vi "Set System Monitor Settings.vi"(8 "error in (no error)":errorcluster, 10 "System Monitor Settings":T1, 11 "Item Ref in":T2 format="%.0x") -> (0 "error out":errorcluster, 3 "Item Ref out":T2 format="%.0x")   [LabVIEW 2027, in "System Monitor System Explorer.lvlib"]
uses:
  System Monitor System Explorer.lvlib
  <vilib>/NI VeriStand/Custom Device API/Custom Device Item Ref.ctl
  Shared/System Monitor Settings.ctl
  Shared/Constants.vi
  <vilib>/NI VeriStand/Custom Device API/Set Item Property (U32).vi
  <vilib>/NI VeriStand/Custom Device API/Set Item Property (Double).vi
  <vilib>/NI VeriStand/Custom Device API/Custom Device API.lvlib
  Shared/System Monitor Shared.lvlib
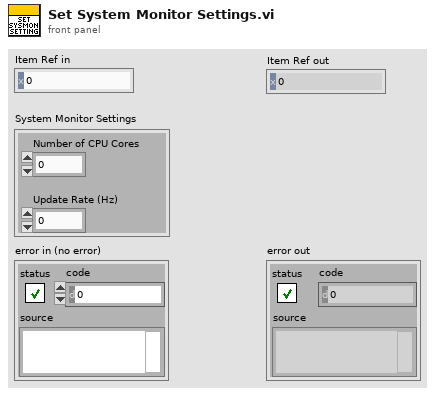
[diagram p1: front panel]
types:
  T1 = typedef "System Monitor Shared.lvlib/System Monitor Settings.ctl" = cluster{"Number of CPU Cores":u64, "Update Rate (Hz)":dbl}
  T2 = typedef "Custom Device API.lvlib/Custom Device Item Ref.ctl" = u64
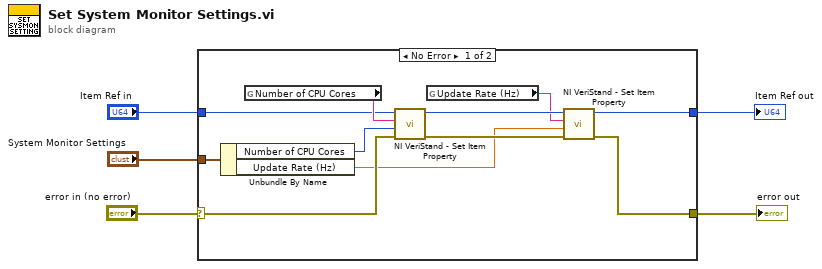
[diagram p0: block diagram]
diagram:
  n1 = case shown="No Error" "error in (no error)" {
    selector: "error in (no error)" -> [w16 w17]
    tunnel: [w9 w17] -> w4
    tunnel: [w10 w18] -> w3
    tunnel: "Item Ref in" -> [w14 w18]
    tunnel: "System Monitor Settings" -> [w8 _]
    frame No Error {
      n2 = Unbundle By Name(w8) -> ("Number of CPU Cores"=w7:u64, "Update Rate (Hz)"=w6:dbl)
      n3 = global read "Constants.vi" "Number of CPU Cores"() -> (w15:string)
      n4 = call-poly <vilib>:"NI VeriStand - Set Item Property.vi"("error in (no error)"=w16, "Value"=w7, "Property Name"=w15, "Item Ref in"=w14) -> ("error out"=w13:errorcluster, "Item Ref out"=w12:T2)  [unwired: 5 in, 1 out]
      n5 = global read "Constants.vi" "Update Rate (Hz)"() -> (w11:string)
      n6 = call-poly <vilib>:"NI VeriStand - Set Item Property.vi"("error in (no error)"=w13, "Value"=w6, "Property Name"=w11, "Item Ref in"=w12) -> ("error out"=w9:errorcluster, "Item Ref out"=w10:T2)  [unwired: 5 in, 1 out]
    }
    frame Error {
    }
  }
  "error out" <- w4
  "Item Ref out" <- w3
